vi "Cache-Broadcast Registry Search Result.vi"(8 "error in (no error)":errorcluster, 10 "JKISM Name":string, 11 "Broadcast state":string) -> (0 "error out":errorcluster, 3 "Array":T3(array[cluster]))   [LabVIEW 2014, in "JKI State Machine++.lvlib"]
uses:
  JKI State Machine++.lvlib
  Typedef/_JKISM_Broadcast_Response_Message_info.ctl
  AdvanceAPI/JKISM++ Broadcast Message Type.ctl
  JKISMQ/_JKISMQFGVOPER.ctl
  Operation-BroadcastRegistry.ctl
  global-Broadcast Cache Change Flag.vi
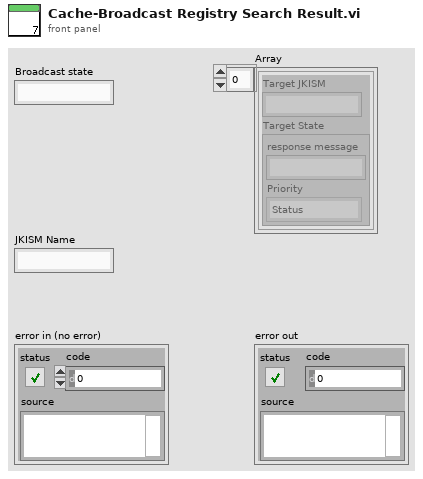
[diagram p1: front panel]
types:
  T1 = typedef "JKI State Machine++.lvlib/_JKISM_Broadcast_Response_Message_info.ctl" = cluster{"response message":string, "Priority":T2}
  T2 = typedef "JKI State Machine++.lvlib/JKISM++ Broadcast Message Type.ctl" = enum16{"Status", "Interrupt(High)"}
  T3 = cluster{"Target JKISM":string, "Target State":T1}[]
  T4 = cluster{"Target JKISM":string, "Target State":T1}
  T5 = typedef "JKI State Machine++.lvlib/_JKISMQFGVOPER.ctl" = enum16{"Get By Name", "List", "Check If Name Exists", "Release", "Module Status"}
  T6 = typedef "JKI State Machine++.lvlib/Operation-BroadcastRegistry.ctl" = enum16{"Delete Source Module", "Delete Target Module", "Remove Module", "Register", "Unregister", "Check"}
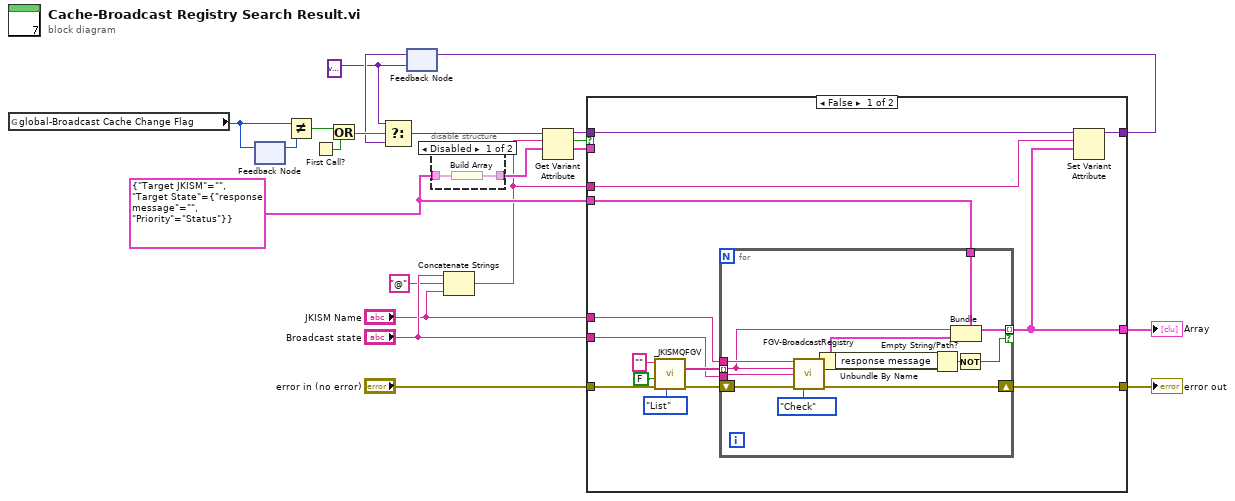
[diagram p0: block diagram]
diagram:
  w9 = T4 {"Target JKISM"="", "Target State"={"response message"="", "Priority"=enum."Status"}} ("cluster")
  w14 = variant
  n1 = global read "global-Broadcast Cache Change Flag.vi" "global-Broadcast Cache Change Flag"() -> (w2:u32)
  n2 = feedback-in #1(w2) -> ()
  n3 = feedback #1() -> (w1:u32)  [unwired: 1 in]
  n4 = Not Equal?(x=w2, y=w1) -> (x != y?=w18:bool)
  n5 = First Call?() -> (First Call?: T/F=w17:bool)
  n6 = Or(x=w18, y=w17) -> (x .or. y?=w16:bool)
  n7 = feedback #2(w14) -> (w15:variant)
  n8 = Select(t=w14, s=w16, f=w15) -> (s? t:f=w10:variant)
  n9 = disable-structure shown="Disabled" {
    disable-tunnel: w9 -> [w23 _]
    disable-tunnel: [w22 _] -> w8
    frame Disabled {
      n10 = Build Array(w23) -> (w22:T3)
    }
    frame Enabled {
    }
  }
  n11 = Concatenate Strings("Broadcast state", "@" ("string"), "JKISM Name") -> (w4:string)
  n12 = Get Variant Attribute(Variant=w10, name=w4, default value (empty Variant)=w8) -> (duplicate Variant=w6:variant, found=w7:bool, value=w5:T3)  [unwired: 1 in, 1 out]
  n13 = case shown="False" w7 {
    tunnel: [w37 w51] -> w21
    tunnel: "error in (no error)" -> [w34 w51]
    tunnel: [w25 w52] -> w19
    tunnel: "Broadcast state" -> [w30 _]
    tunnel: "JKISM Name" -> [w29 _]
    tunnel: w9 -> [w28 _]
    tunnel: w6 -> [w27 w50]
    tunnel: w5 -> [_ w52]
    tunnel: w4 -> [w26 _]
    tunnel: [w24 w50] -> w3
    frame False {
      n14 = call "_JKISMQFGV.vi"(6:_JKISMQFGVOPER."List", "Error in"=w34, "create if not found? (T)"=FALSE, "Name(\"\" to use uuid) in"="" ("Name(\"\" to use uuid) in")) -> ("Error out"=w36:errorcluster, "Name"=w35:string[])  [unwired: 4 in, 2 out]
      n15 = for {
        tunnel: w35 -> [w44] mode=indexing
        tunnel: w29 -> [w47]
        tunnel: w30 -> [w42]
        shift-right: [w45] -> w37
        shift-left: w36 -> [w48]
        tunnel: [w41] -> w25 mode=indexing if=w43
        tunnel: w28 -> [w39]
        n16 = call "FGV-BroadcastRegistry.vi"("Source"=w47, "Target"=w44, "Message"=w42, "Error in"=w48, "Operation"=Operation-BroadcastRegistry."Check") -> ("Response Message Info"=w40:T1, "Error out"=w45:errorcluster)  [unwired: 8 in, 1 out]
        n17 = Unbundle By Name(w40) -> ("response message"=w38:string)
        n18 = Empty String/Path?(string/path=w38) -> (empty?=w46:bool)
        n19 = Bundle(cluster=w39, "Target JKISM"=w44, "Target State"=w40) -> (w41:T4)
        n20 = Not(x=w46) -> (.not. x?=w43:bool)
      }
      n21 = Set Variant Attribute(Variant=w27, name=w26, value=w25) -> (Variant out=w24:variant)  [unwired: 1 in, 2 out]
    }
    frame True {
    }
  }
  "error out" <- w21
  "Array" <- w19
  n22 = feedback-in #2(w3) -> ()
